vi "captureTopBottomExp.vi"(8 "error in (no error)":errorcluster, 10 "Array in":refnum<k7>[](array[refnum]), 11 "Cluster in":refnum<vi>) -> (0 "error out":errorcluster, 3 "Value":T1)   [LabVIEW 2014]
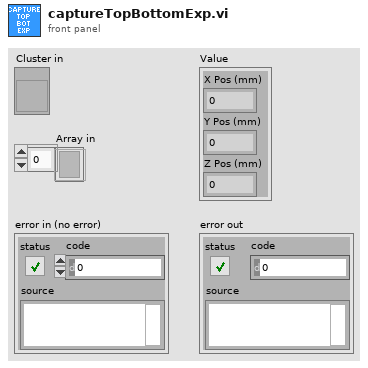
[diagram p1: front panel]
types:
  T1 = cluster{"X Pos (mm)":sgl, "Y Pos (mm)":sgl, "Z Pos (mm)":sgl}
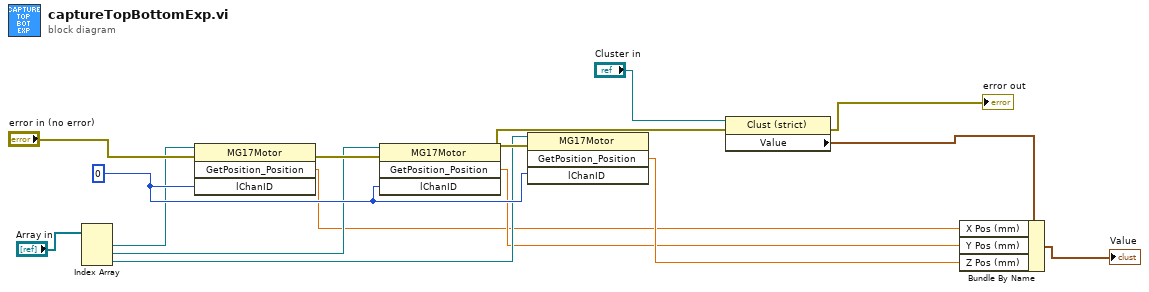
[diagram p0: block diagram]
diagram:
  w12 = 0 ("lChanID")
  n1 = Index Array(array="Array in") -> (element #1=w3:refnum<k7>, element #2=w5:refnum<k7>, element #3=w7:refnum<k7>)  [unwired: 3 in]
  n2 = invoke class="MG17Motor" method="GetPosition_Position"(reference=w3, error in="error in (no error)", "lChanID"=w12) -> (error out=w15:errorcluster, "GetPosition_Position"=w4:sgl)  [unwired: 1 in, 2 out]
  n3 = invoke class="MG17Motor" method="GetPosition_Position"(reference=w5, error in=w15, "lChanID"=w12) -> (error out=w16:errorcluster, "GetPosition_Position"=w6:sgl)  [unwired: 1 in, 2 out]
  n4 = invoke class="MG17Motor" method="GetPosition_Position"(reference=w7, error in=w16, "lChanID"=w12) -> (error out=w9:errorcluster, "GetPosition_Position"=w8:sgl)  [unwired: 1 in, 2 out]
  n5 = property on="Property Node" class="Clust (strict)"(reference="Cluster in", error in=w9) -> (error out=→"error out":errorcluster, "Value"=w10:T1)  [unwired: 1 out]
  n6 = Bundle By Name(cluster=w10, "X Pos (mm)"=w4, "Y Pos (mm)"=w6, "Z Pos (mm)"=w8) -> (→"Value":T1)
